vi "FMDLConfigKeithley6514AmmeterModeTriggered.vi"(6 "Arm Timer Interval (0.1 s)":dbl=0.1, 7 "Integration Time (1 PLCs)":dbl=1.0, 8 "error in (no error)":errorcluster, 9 "Arm Count (1)":i32=1, 10 "Arm Source (1: Immediate)":i32(ring)=1 items=["Hold", "Immediate", "Real-time Clock", "Manual", "Bus", "Trigger Link", "External Triggering", "Timer", "STest", "PSTest", "NSTest", "BSTest"], 11 "VISA resource name":refnum<visa-resource-name>) -> (0 "error out":errorcluster, 3 "VISA resource name out":refnum<visa-resource-name>)   [LabVIEW 2018]
uses:
  <instrlib>/Keithley 6517/Keithley 6517.lvlib
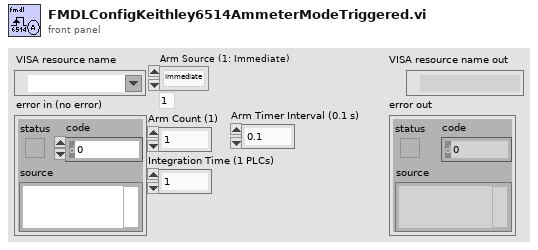
[diagram p1: front panel]
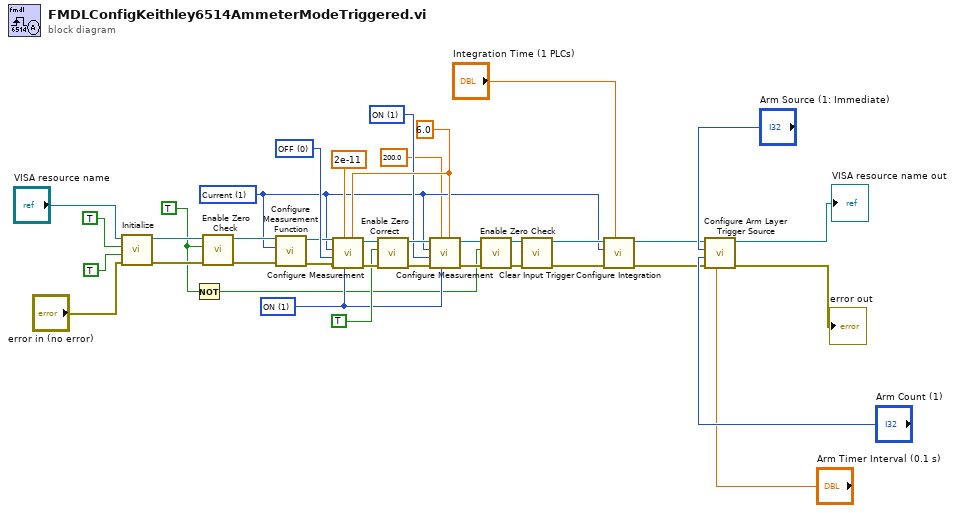
[diagram p0: block diagram]
diagram:
  w24 = 6.0 ("Display Resolution (6)")
  w15 = 1 items=["OFF", "ON", "ONCE"] ("Auto Range (1: ON)")
  w25 = 1 items=["OFF", "ON", "ONCE"] ("Auto Resolution (1: ON)")
  w34 = 0 items=["OFF", "ON", "ONCE"] ("Auto Range (1: ON)")
  w3 = 1 items=["Voltage", "Current", "Resistance", "Charge"] ("Measurement Function (0: Voltage)")
  w21 = TRUE ("Enable Zero Check (T: Enable)")
  n1 = call <instrlib>:"Initialize.vi"("error in (no error)"="error in (no error)", "Reset (True)"=TRUE, "ID Query (True)"=TRUE, "VISA resource name"="VISA resource name") -> ("error out"=w38:errorcluster, "VISA resource name out"=w37:refnum<visa-resource-name>)  [unwired: 6 in]
  n2 = Not(x=w21) -> (.not. x?=w20:bool)
  n3 = call <instrlib>:"Enable Zero Check.vi"("error in (no error)"=w38, "Enable Zero Check (T: Enable)"=w21, "VISA resource name"=w37) -> ("error out"=w36:errorcluster, "VISA resource name out"=w35:refnum<visa-resource-name>)  [unwired: 7 in]
  n4 = call <instrlib>:"Configure Measurement Function.vi"("error in (no error)"=w36, "Measurement Function (0: Voltage)"=w3, "VISA resource name"=w35) -> ("error out"=w32:errorcluster, "VISA resource name out"=w33:refnum<visa-resource-name>)  [unwired: 7 in]
  n5 = call <instrlib>:"Configure Measurement.vi"("Display Resolution (6)"=w24, "Auto Resolution (1: ON)"=w25, "Auto Range Value (2.0000000E+2)"=2e-11, "error in (no error)"=w32, "Auto Range (1: ON)"=w34, "Measurement Function (0: Voltage)"=w3, "VISA resource name"=w33) -> ("error out"=w31:errorcluster, "VISA resource name out"=w30:refnum<visa-resource-name>)  [unwired: 3 in]
  n6 = call <instrlib>:"Enable Zero Correct.vi"("error in (no error)"=w31, "Enable Zero Correct (F: Disable)"=TRUE, "VISA resource name"=w30) -> ("error out"=w27:errorcluster, "VISA resource name out"=w28:refnum<visa-resource-name>)  [unwired: 7 in]
  n7 = call <instrlib>:"Configure Measurement.vi"("Display Resolution (6)"=w24, "Auto Resolution (1: ON)"=w25, "Auto Range Value (2.0000000E+2)"=200.0, "error in (no error)"=w27, "Auto Range (1: ON)"=w15, "Measurement Function (0: Voltage)"=w3, "VISA resource name"=w28) -> ("error out"=w22:errorcluster, "VISA resource name out"=w23:refnum<visa-resource-name>)  [unwired: 3 in]
  n8 = call <instrlib>:"Enable Zero Check.vi"("error in (no error)"=w22, "Enable Zero Check (T: Enable)"=w20, "VISA resource name"=w23) -> ("error out"=w14:errorcluster, "VISA resource name out"=w13:refnum<visa-resource-name>)  [unwired: 7 in]
  n9 = call <instrlib>:"Clear Input Trigger.vi"("error in (no error)"=w14, "VISA resource name"=w13) -> ("error out"=w5:errorcluster, "VISA resource name out"=w7:refnum<visa-resource-name>)  [unwired: 8 in]
  n10 = call <instrlib>:"Configure Integration.vi"("Integration Time (1 PLCs)"="Integration Time (1 PLCs)", "error in (no error)"=w5, "Measurement Function (0: Voltage)"=w3, "VISA resource name"=w7) -> ("error out"=w4:errorcluster, "VISA resource name out"=w6:refnum<visa-resource-name>)  [unwired: 6 in]
  n11 = call <instrlib>:"Configure Arm Layer Trigger Source.vi"("Arm Timer Interval (0.1 s)"="Arm Timer Interval (0.1 s)", "error in (no error)"=w4, "Arm Count (1)"="Arm Count (1)", "Arm Source (1: Immediate)"="Arm Source (1: Immediate)", "VISA resource name"=w6) -> ("error out"=→"error out":errorcluster, "VISA resource name out"=→"VISA resource name out":refnum<visa-resource-name>)  [unwired: 5 in]
